vi "createCamera.vi"(8 "error in":errorcluster, 10 "Camera":string="ProEM_WinX32") -> (0 "error out":errorcluster, 3 "cameraObj":string)   [LabVIEW 2009]
uses:
  Hal/Channels/Camera/Camera/Camera.lvclass
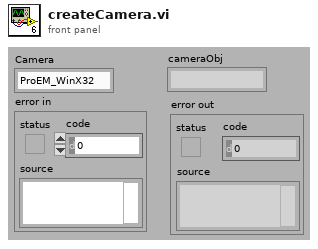
[diagram p1: front panel]
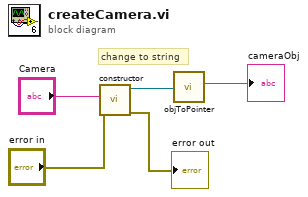
[diagram p0: block diagram]
diagram:
  # "change to string"
  n1 = call "constructor.vi"("error in (no error)"="error in", "Camera"="Camera") -> ("error out"=→"error out":errorcluster, "Camera out"=w2:refnum<class "Camera.lvclass">)  [unwired: 8 in]
  n2 = call "objToPointer.vi"("objIn"=w2) -> ("stringOut"=→"cameraObj":string)  [unwired: 10 in]
